vi "Global 2.vi"() -> ()   [LabVIEW 2010]
panel:
  in  "Groups":string="贤:市"
  in  "sch_per":i32=30 caption="Периодичность опроса, мин" min=1 max=600 format="%#.0f"
  in  "restart":bool=TRUE caption="Перезагрузка\nпо ошибке PXI"
  in  "KR_data":string="ssh.alwaysdata.com:12673" caption="Сервер данных КР"
  in  "schedule":bool caption="Расписание?"
  in  "StartPath":path=path "C:/skil/skil" caption="Путь запуска"
  in  "Ver":string caption="Версия"
  in  "send":bool caption="Отправлять?"
  in  "save":bool caption="Сохранять?"
  in  "SMGR_link":string="http://smgr.alwaysdata.net/post_event/" caption="Сервер данных РГПН"
  in  "DevNo":i32=14 caption="Измеритель №"
  in  "ch":T1(array[cluster])=[{"name"=enum."sync", "num"=3, "Numeric"=0}, {"name"=enum."phase_a", "num"=1, "Numeric"=0}, {"name"=enum."phase_b", "num"=0, "Numeric"=0}, {"name"=enum."phase_c", "num"=2, "Numeric"=0}] caption="Каналы АЦП"
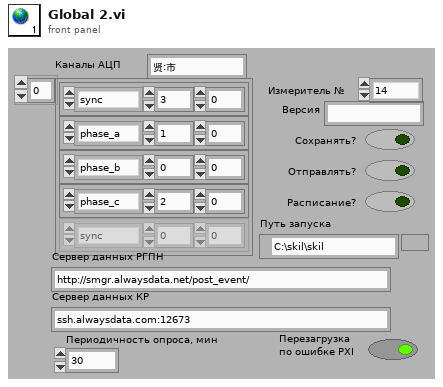
[diagram p1: front panel]
types:
  T1 = cluster{"name":enum16{"sync", "phase_a", "phase_b", "phase_c", "ground"}, "num":i32, "Numeric":i32}[]
diagram:
